vi "Check for Timeout Error.vi"(8 "error in (no error)":errorcluster, 10 "Timeout (10000ms)":u32=10000, 11 "t0":u32) -> (0 "error out":errorcluster)   [LabVIEW 2013, in "OpenSSL Socket.lvlib" / "SSL-Lib.lvclass"]
uses:
  SSL-Lib.lvclass
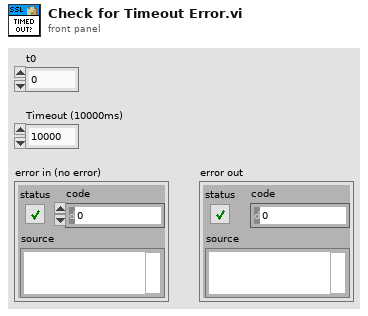
[diagram p1: front panel]
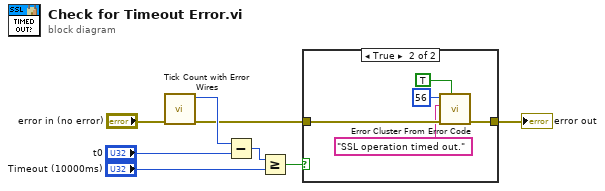
[diagram p0: block diagram]
diagram:
  n1 = call "Tick Count with Error Wires.vi"("error in (no error)"="error in (no error)") -> ("error out"=w2:errorcluster, "millisecond timer value"=w5:u32)  [unwired: 9 in]
  n2 = Subtract(x=w5, y="t0") -> (x-y=w7:u32)
  n3 = Greater Or Equal?(x=w7, y="Timeout (10000ms)") -> (x >= y?=w3:bool)
  n4 = case shown="True" w3 {
    tunnel: w2 -> [w9 w13]
    tunnel: [w9 w14] -> w1
    frame False {
    }
    frame True {
      n5 = call <vilib>:"Error Cluster From Error Code.vi"("show call chain? (False)"=TRUE, "error in (no error)"=w13, "error message (\"\")"="SSL operation timed out." ("error message (\"\")"), "error code (0)"=56) -> ("error out"=w14:errorcluster)  [unwired: 5 in]
    }
  }
  "error out" <- w1
